vi "325 Configure setpoint text.vi"() -> ()   [LabVIEW 2019, in "nematic.lvlib"]
uses:
  nematic.lvlib
  lib/Lake Shore 325/Lake Shore 325.lvlib
panel:
  out "error out 2":errorcluster
  out "VISA resource name out 2":refnum<visa-resource-name>
  in  "Rate Value (0.0)":dbl format="%.1f"
  out "Sensor Data 2":dbl format="%.4f"
  in  "error in (no error) 2":errorcluster
  in  "VISA Refnum in 2":refnum<visa-resource-name>
  in  "Sensor Input (0:A)":u16(ring) items=["A", "B"]
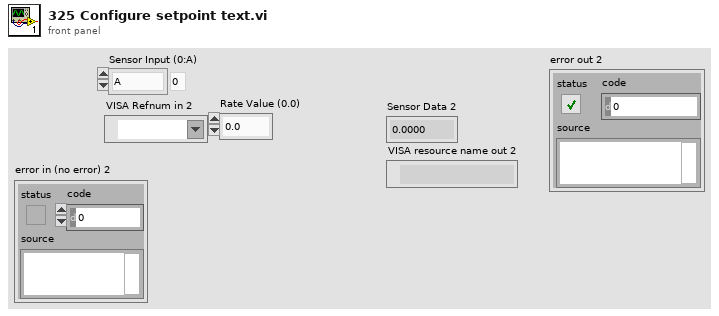
[diagram p1: front panel]
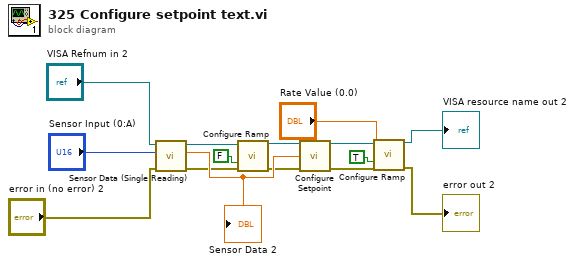
[diagram p0: block diagram]
diagram:
  n1 = call "Sensor Data (Single Reading).vi"("error in (no error)"="error in (no error) 2", "Sensor Input (0:A)"="Sensor Input (0:A)", "VISA resource name"="VISA Refnum in 2") -> ("error out"=w6:errorcluster, "Sensor Data"=w10:dbl, "VISA resource name out"=w13:refnum<visa-resource-name>)  [unwired: 6 in]
  "Sensor Data 2" <- w10
  n2 = call "Configure Ramp.vi"("VISA resource name"=w13, "Setpoint Ramp (F: Off)"=FALSE, "error in (no error)"=w6) -> ("VISA resource name out"=w11:refnum<visa-resource-name>, "error out"=w5:errorcluster)  [unwired: 11 in]
  n3 = call "Configure Setpoint.vi"("VISA resource name"=w11, "Setpoint Value (0.0000)"=w10, "error in (no error)"=w5) -> ("VISA resource name out"=w9:refnum<visa-resource-name>, "error out"=w4:errorcluster)  [unwired: 11 in]
  n4 = call "Configure Ramp.vi"("VISA resource name"=w9, "Rate Value (0.0)"="Rate Value (0.0)", "Setpoint Ramp (F: Off)"=TRUE, "error in (no error)"=w4) -> ("VISA resource name out"=→"VISA resource name out 2":refnum<visa-resource-name>, "error out"=→"error out 2":errorcluster)  [unwired: 10 in]
